vi "Geracao_Excel.vi"(8 "error in (no error)":errorcluster, 11 "FileName":string caption="NomeDocumento") -> (0 "error out":errorcluster)   [LabVIEW 2019]
uses:
  0a471edf-c676-4e06-b2ff-6746a7f8de60.vi
  SalvarDadosTemporario.vi
  TelaConfig/Configuracao.Variaveis.vi
  <vilib>/Utility/file.llb/Write Delimited Spreadsheet (string).vi
panel:
  out "Cluster":T1={"Graph"=[], "Data"=timestamp(3705620400 s since 1904-01-01), "ModeloMotor"="", "ModeloInversor"="", "ModeloAeroGerador"="", "PotenciaAero"=""}
  out "PathMeasure":path
  out "SavedList":string[][](array[string])
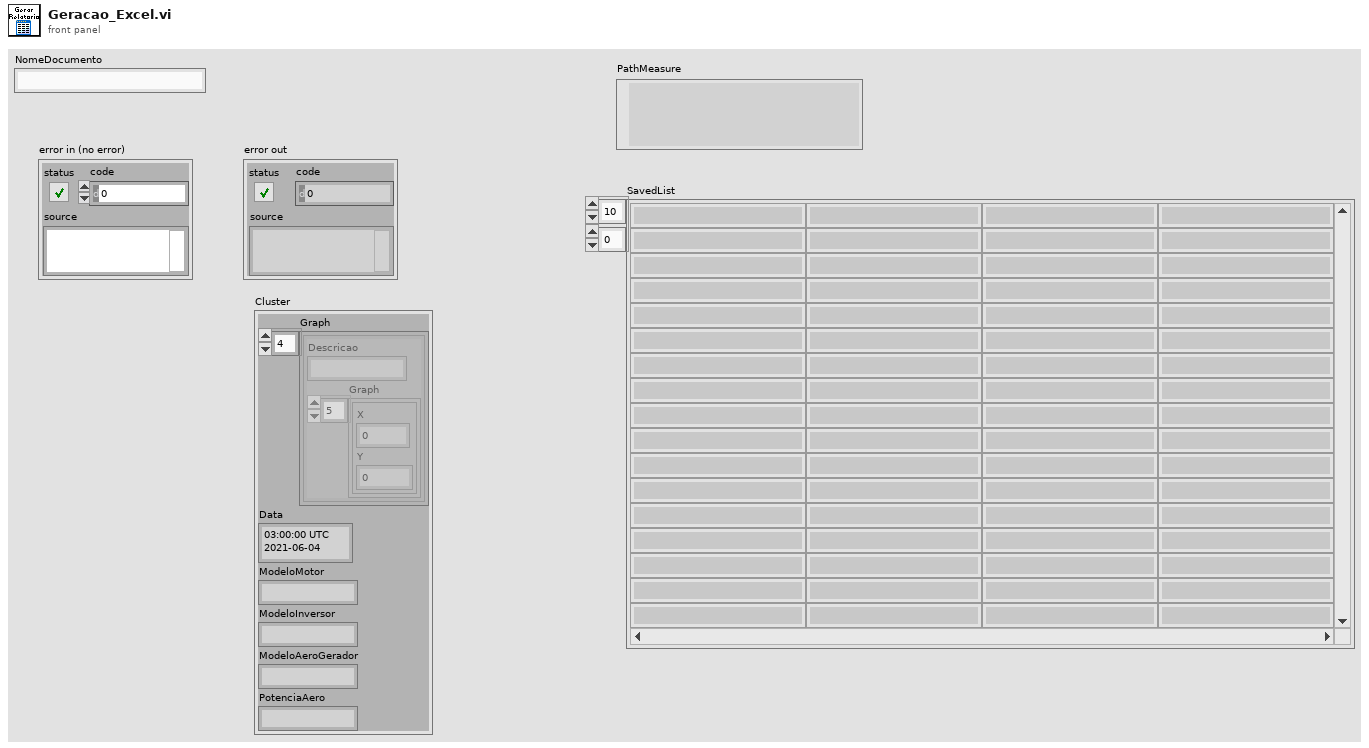
[diagram p1: front panel]
types:
  T1 = cluster{"Graph":cluster{"Descricao":string, "Graph":cluster{"X":dbl, "Y":dbl}[]}[], "Data":timestamp, "ModeloMotor":string, "ModeloInversor":string, "ModeloAeroGerador":string, "PotenciaAero":string}
  T2 = cluster{"Descricao":string, "Graph":cluster{"X":dbl, "Y":dbl}[]}[]
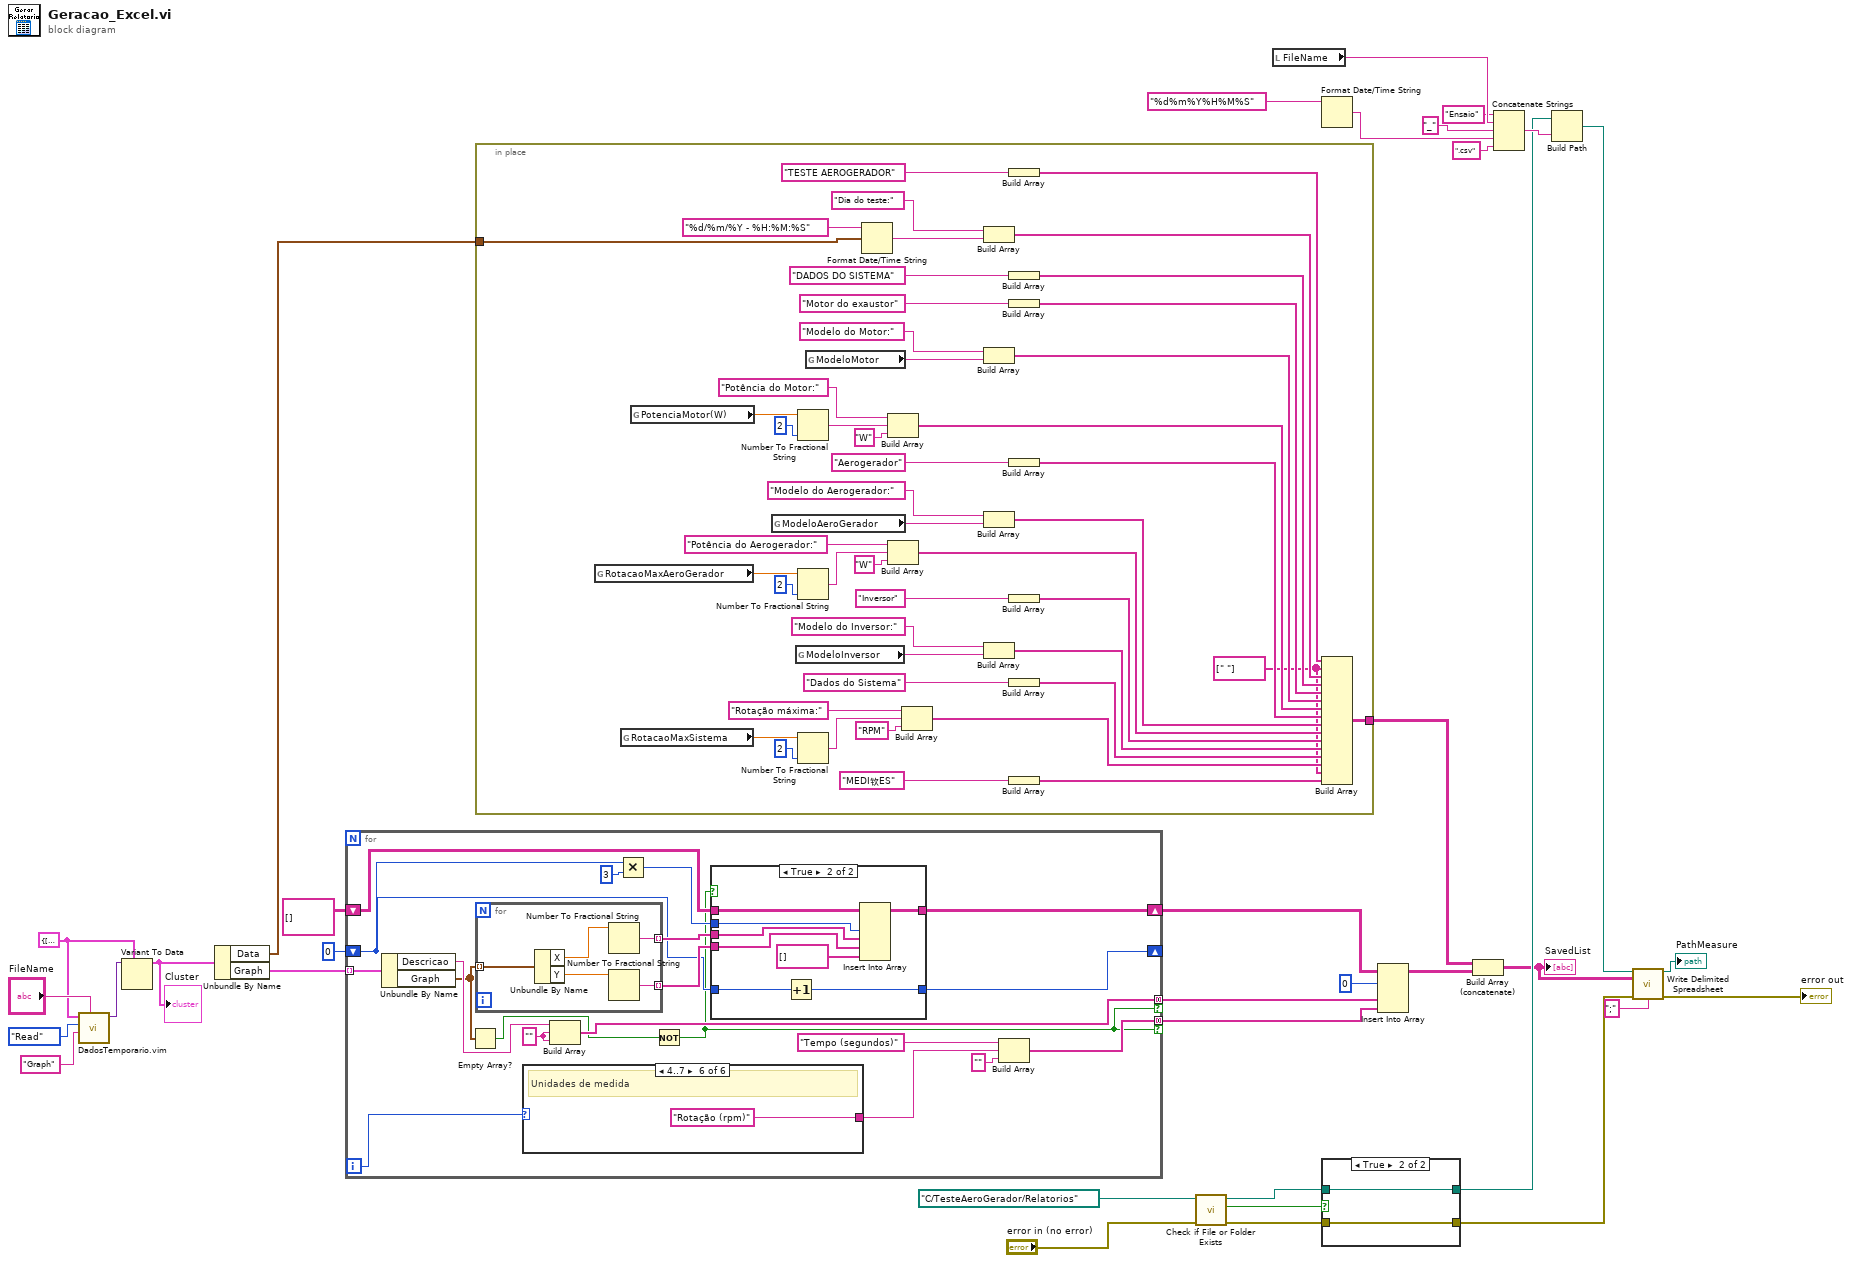
[diagram p0: block diagram]
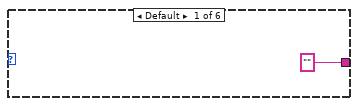
[diagram p3: hidden frame]
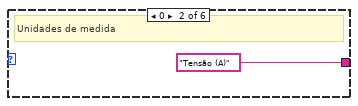
[diagram p4: hidden frame]
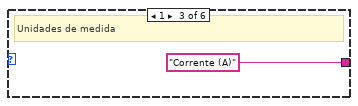
[diagram p5: hidden frame]
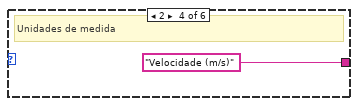
[diagram p6: hidden frame]
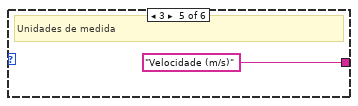
[diagram p7: hidden frame]
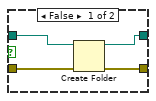
[diagram p8: hidden frame]
diagram:
  w17 = T1 {"Graph"=[], "Data"=timestamp(3705620400 s since 1904-01-01), "ModeloMotor"="", "ModeloInversor"="", "ModeloAeroGerador"="", "PotenciaAero"=""} ("Cluster")
  n1 = call "DadosTemporario.vim"("FileName"="FileName", "Directory"="Graph", "Read/Write(Read)"=enum16{"Read", "Write"}."Read", "DataInp"=w17) -> ("DataOut"=w16:variant)  [unwired: 6 in, 1 out]
  n2 = Variant To Data(type=w17, Variant=w16) -> (data=w14:T1)  [unwired: 1 in, 1 out]
  "Cluster" <- w14
  n3 = Unbundle By Name(w14) -> ("Data"=w15:timestamp, "Graph"=w13:T2)
  n4 = for {
    tunnel: w13 -> [w55] mode=indexing
    shift-right: [w47] -> w9
    shift-left: string[][] [] -> [w48]
    tunnel: [w46] -> w10 mode=concatenating if=w37
    tunnel: [w42] -> w8 mode=concatenating if=w37
    shift-right: [w39] -> _
    shift-left: 0 -> [w38]
    i -> [w36]
    w53 = ""
    n5 = Unbundle By Name(w55) -> ("Descricao"=w54:string, "Graph"=w41:cluster{"X":dbl, "Y":dbl}[])
    n6 = Empty Array?(array=w41) -> (empty?=w40:bool)
    n7 = for {
      tunnel: w41 -> [w76] mode=indexing
      tunnel: [w73] -> w50 mode=indexing
      tunnel: [w72] -> w49 mode=indexing
      n8 = Unbundle By Name(w76) -> ("X"=w75:dbl, "Y"=w74:dbl)
      n9 = Number To Fractional String(number=w75) -> (F-format string=w73:string)  [unwired: 3 in]
      n10 = Number To Fractional String(number=w74) -> (F-format string=w72:string)  [unwired: 3 in]
    }
    n11 = case shown="4..7" w36 {
      tunnel: ["" "Tensão (A)" "Corrente (A)" "Velocidade (m/s)" "Velocidade (m/s)" "Rotação (rpm)"] -> w45
      frame Default {
      }
      frame 0 {
        # "Unidades de medida"
      }
      frame 1 {
        # "Unidades de medida"
      }
      frame 2 {
        # "Unidades de medida"
      }
      frame 3 {
        # "Unidades de medida"
      }
      frame 4..7 {
        # "Unidades de medida"
      }
    }
    n12 = Build Array(w54, w53, w53) -> (w46:string[])
    n13 = Multiply(x=w38, y=3) -> (x*y=w51:i32)
    n14 = Not(x=w40) -> (.not. x?=w37:bool)
    n15 = case shown="True" w37 {
      tunnel: w51 -> [_ w65]
      tunnel: w50 -> [_ w64]
      tunnel: w49 -> [_ w63]
      tunnel: w48 -> [w57 w62]
      tunnel: [w57 w61] -> w47
      tunnel: w38 -> [w56 w59]
      tunnel: [w56 w58] -> w39
      frame False {
      }
      frame True {
        n16 = Increment(x=w59) -> (x+1=w58:i32)
        n17 = Insert Into Array(array=w62, index (col)=w65, new element #1=w64, new element #2=w63, new element #3=string[] [] ("new element/subarray")) -> (w61:string[][])  [unwired: 1 in]
      }
    }
    n18 = Build Array("Tempo (segundos)" ("element"), w45, "" ("element")) -> (w42:string[])
  }
  n19 = in-place {
    in-place-border: w15 -> [w87]
    in-place-border: [w77] -> w6
    w80 = string[] [" "]
    n20 = global read "Configuracao.Variaveis.vi" "RotacaoMaxAeroGerador"() -> (w111:dbl)
    n21 = global read "Configuracao.Variaveis.vi" "RotacaoMaxSistema"() -> (w106:dbl)
    n22 = global read "Configuracao.Variaveis.vi" "PotenciaMotor(W)"() -> (w122:dbl)
    n23 = global read "Configuracao.Variaveis.vi" "ModeloAeroGerador"() -> (w110:string)
    n24 = global read "Configuracao.Variaveis.vi" "ModeloInversor"() -> (w107:string)
    n25 = Number To Fractional String(number=w122, precision (6)=i16 2) -> (F-format string=w120:string)  [unwired: 2 in]
    n26 = Number To Fractional String(number=w111, precision (6)=i16 2) -> (F-format string=w113:string)  [unwired: 2 in]
    n27 = Number To Fractional String(number=w106, precision (6)=i16 2) -> (F-format string=w104:string)  [unwired: 2 in]
    n28 = global read "Configuracao.Variaveis.vi" "ModeloMotor"() -> (w123:string)
    n29 = Format Date/Time String(time format string (%c)="%d/%m/%Y - %H:%M:%S", seconds (now)=w87) -> (date/time string=w89:string)  [unwired: 1 in]
    n30 = Build Array("Potência do Motor:", w120, "W" ("element")) -> (w116:string[])
    n31 = Build Array("Potência do Aerogerador:", w113, "W" ("element")) -> (w95:string[])
    n32 = Build Array("Rotação máxima:", w104, "RPM" ("element")) -> (w91:string[])
    n33 = Build Array("Dia do teste:", w89) -> (w88:string[])
    n34 = Build Array("Modelo do Motor:", w123) -> (w117:string[])
    n35 = Build Array("Modelo do Aerogerador:", w110) -> (w96:string[])
    n36 = Build Array("Modelo do Inversor:", w107) -> (w93:string[])
    n37 = Build Array("TESTE AEROGERADOR") -> (w84:string[])
    n38 = Build Array("DADOS DO SISTEMA") -> (w81:string[])
    n39 = Build Array("Motor do exaustor") -> (w83:string[])
    n40 = Build Array("Aerogerador") -> (w97:string[])
    n41 = Build Array("Inversor") -> (w94:string[])
    n42 = Build Array("Dados do Sistema") -> (w92:string[])
    n43 = Build Array("MEDI钦ES") -> (w78:string[])
    n44 = Build Array(w84, w80, w88, w81, w83, w117, w116, w97, w96, w95, w94, w93, w92, w91, w80, w78) -> (w77:string[][])
  }
  n45 = call <vilib>:"Check if File or Folder Exists.vi"("error in (no error)"="error in (no error)", "path"=path "C:/TesteAeroGerador/Relatorios" ("file path (dialog if empty)")) -> ("error out"=w26:errorcluster, "file or folder exists?"=w27:bool, "dup path"=w25:path)  [unwired: 7 in]
  n46 = local read "FileName"() -> (w3:string)
  n47 = Format Date/Time String(time format string (%c)="%d%m%Y%H%M%S") -> (date/time string=w31:string)  [unwired: 2 in]
  n48 = case shown="True" w27 {
    tunnel: w26 -> [w128 w130]
    tunnel: [w125 w130] -> w22
    tunnel: [w126 w129] -> w23
    tunnel: w25 -> [w127 w129]
    frame False {
      n49 = Create Folder(path (use dialog)=w127, error in=w128) -> (created path=w126:path, error out=w125:errorcluster)  [unwired: 1 in, 1 out]
    }
    frame True {
    }
  }
  n50 = Insert Into Array(array=w9, index (row)=0, new element #1=w10, new element #2=w8) -> (w5:string[][])  [unwired: 1 in]
  n51 = Build Array (concatenate)(w6, w5) -> (w4:string[][])
  "SavedList" <- w4
  n52 = Concatenate Strings("Ensaio" ("string"), w3, "_" ("string"), w31, ".csv" ("string")) -> (w35:string)
  n53 = Build Path(base path=w23, name or relative path=w35) -> (appended path=w30:path)
  n54 = call-poly <vilib>:"Write Delimited Spreadsheet.vi"("file path (dialog if empty)"=w30, "2D data"=w4, "error in (no error)"=w22, "delimiter (\\t)"=";" ("delimiter (\\t)")) -> ("new file path (Not A Path if cancelled)"=→"PathMeasure":path, "error out"=→"error out":errorcluster)  [unwired: 10 in]
